vi "Untitled 1.vi"() -> ()   [LabVIEW 2019]
uses:
  <vilib>/Analysis/Matrix/NI_Matrix.lvlib
  <vilib>/Analysis/Matrix/Numeric/Add/Add - RM,RM.vi
  <vilib>/Analysis/Matrix/Datatypes/RealMatrix.ctl
panel:
  in  "Real Matrix 2":T1
  in  "Real Matrix":T1
  out "matrice":bool[][](array[boolean])
  in  "vect":dbl[](array[numeric])
  out "NB ITERATIONS":i32
  in  "STOP":bool
  out "x*y":dbl
  in  "stop":bool
  out "TE(ms)":u32
  out "TF(ms)":dbl
  out "IT(ms)":dbl
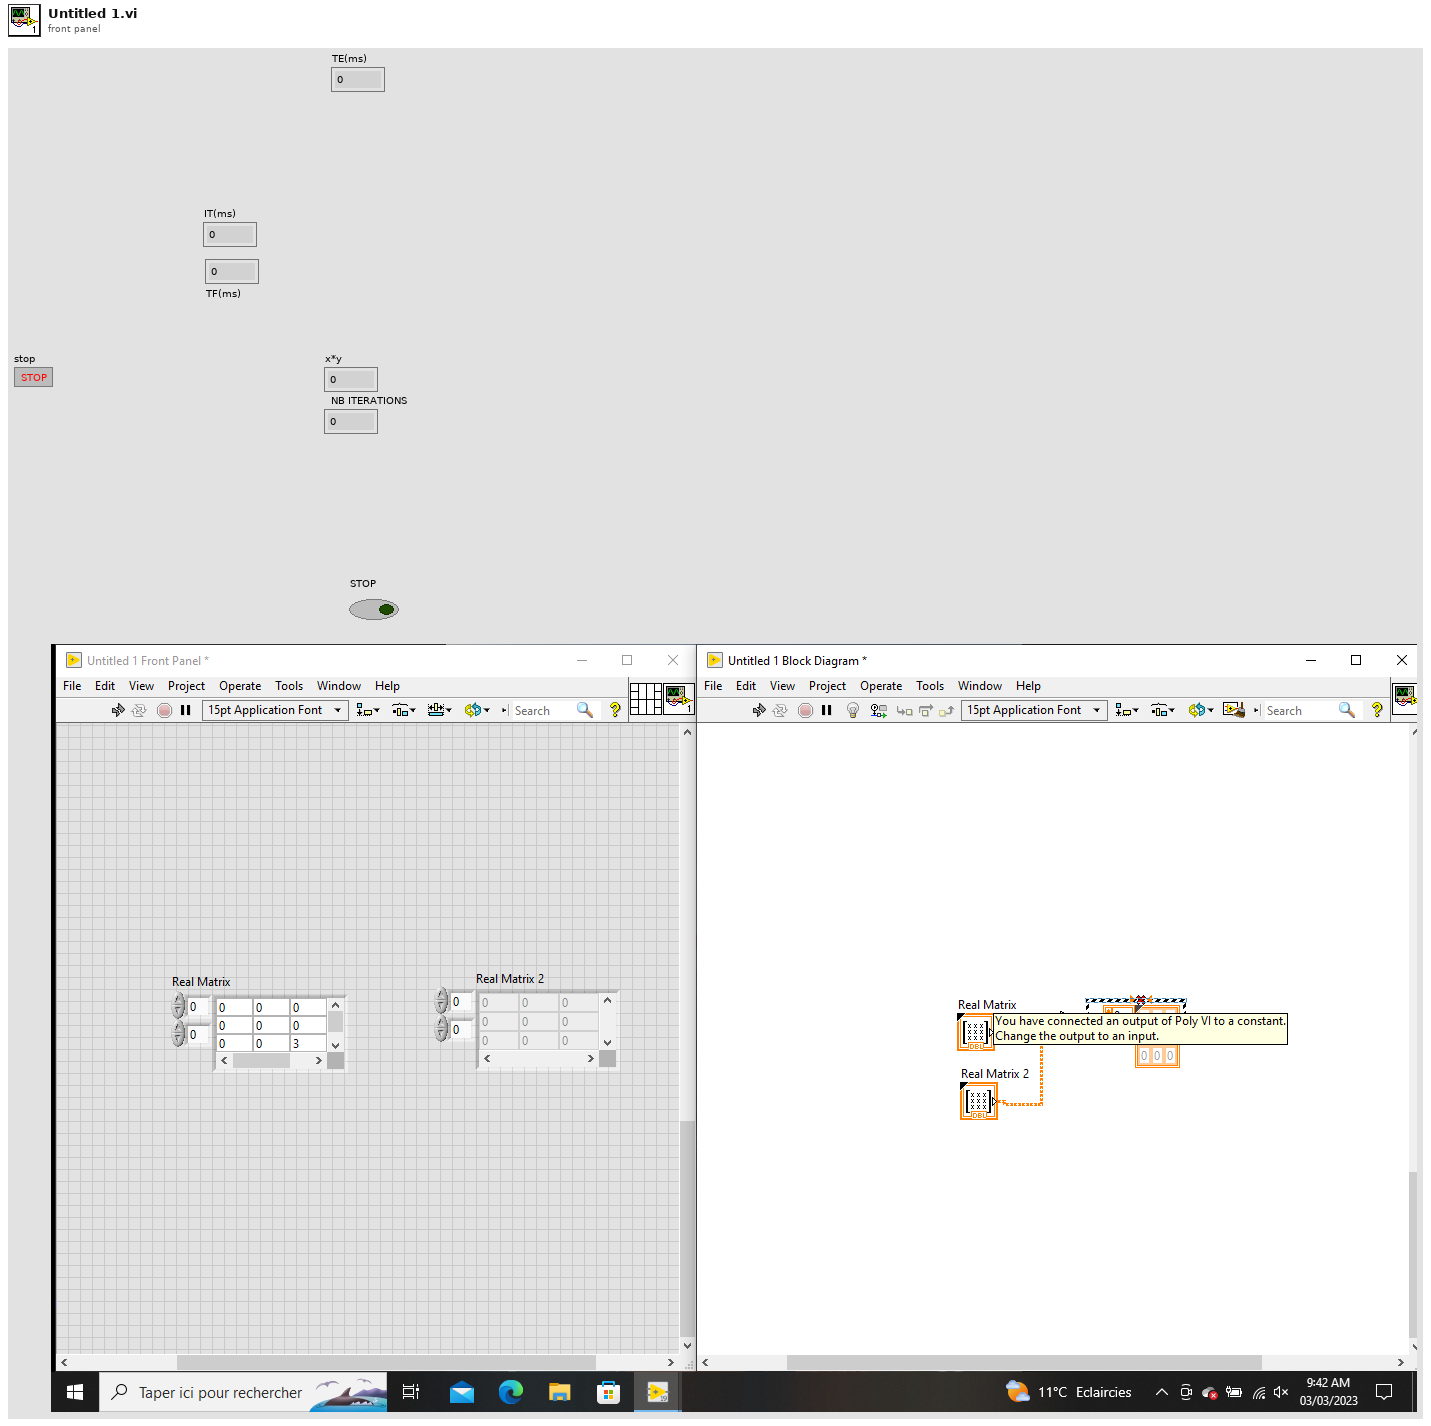
[diagram p1: front panel]
types:
  T1 = typedef "NI_Matrix.lvlib/RealMatrix.ctl" = dbl[][]
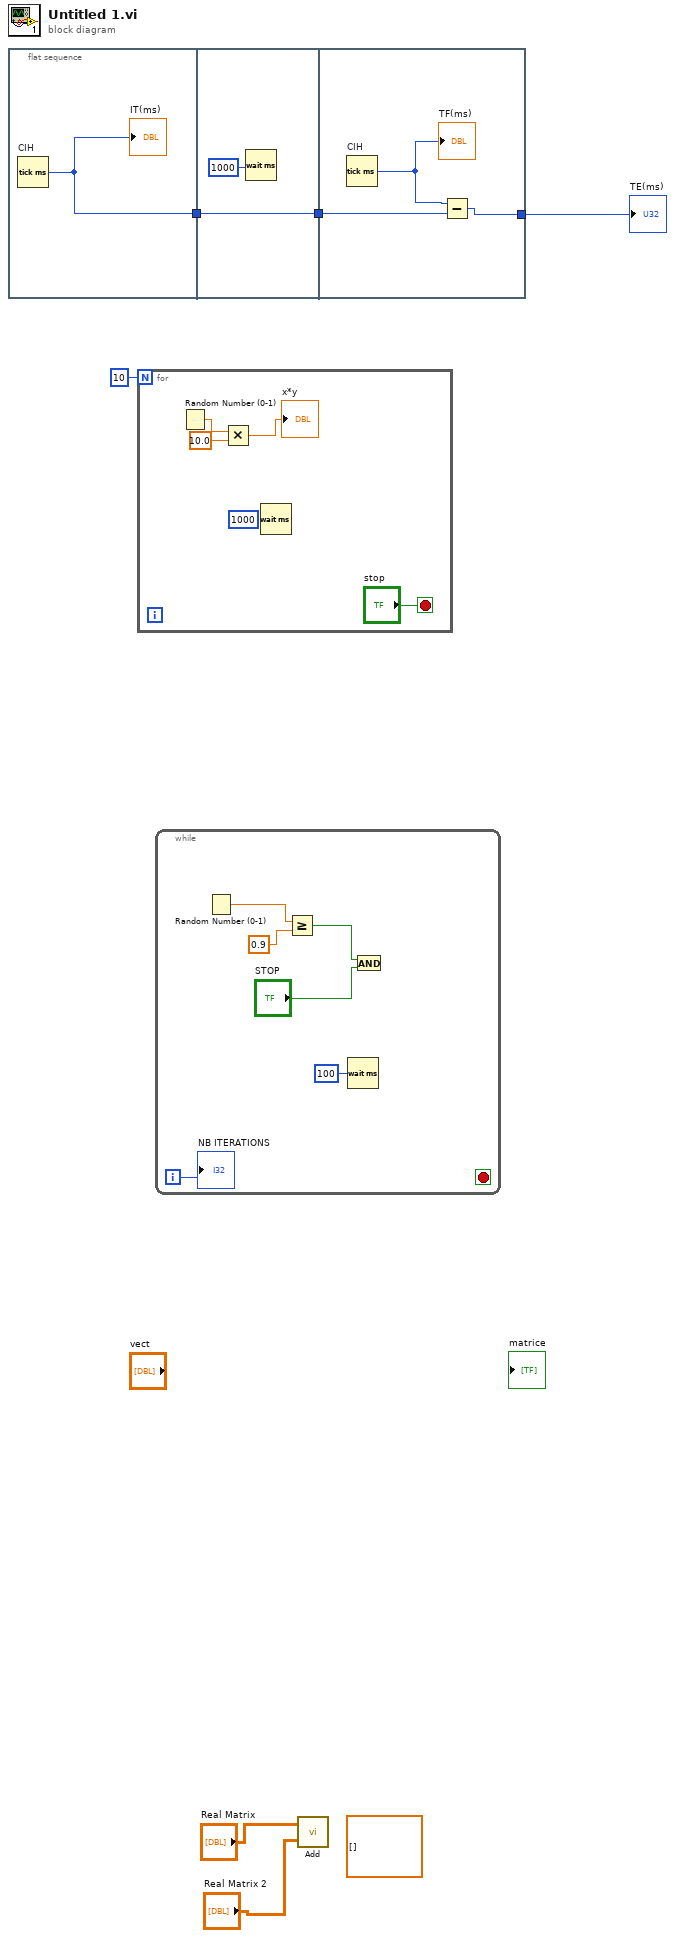
[diagram p0: block diagram]
diagram:
  (unwired) T1 [] ("Real Matrix B")
  n1 = flat-sequence {
    tunnel: [w7] -> w5
    tunnel: [w9] -> w6
    tunnel: w5 -> [w9]
    tunnel: w6 -> [w12]
    tunnel: [w10] -> w4
    frame #0 {
      n2 = Tick Count (ms) "CIH"() -> (millisecond timer value=w7:u32)
      "IT(ms)" <- w7
    }
    frame #1 {
      n3 = Wait (ms)(milliseconds to wait=u32 1000 ("millisecond timer value")) -> ()  [unwired: 1 out]
    }
    frame #2 {
      n4 = Tick Count (ms) "CIH"() -> (millisecond timer value=w11:u32)
      "TF(ms)" <- w11
      n5 = Subtract(x=w11, y=w12) -> (x-y=w10:u32)
    }
  }
  n6 = for {
    N: 10 -> [_]
    stop <- "stop" stop-if-true
    (unwired) u32 1000 ("millisecond timer value")
    n7 = Random Number (0-1)() -> (number: 0 to 1=w16:dbl)
    n8 = Multiply(x=w16, y=10.0) -> (x*y=→"x*y":dbl)
    n9 = Wait (ms)() -> ()  [unwired: 1 in, 1 out]
  }
  n10 = while {
    i -> [w20]
    stop <- _ stop-if-true
    n11 = Random Number (0-1)() -> (number: 0 to 1=w18:dbl)
    n12 = Greater Or Equal?(x=w18, y=0.9 ("x")) -> (x >= y?=w21:bool)
    n13 = Wait (ms)(milliseconds to wait=u32 100) -> ()  [unwired: 1 out]
    n14 = And(x=w21, y="STOP") -> ()  [unwired: 1 out]
    "NB ITERATIONS" <- w20
  }
  n15 = call-poly <vilib>:"Add.vi"("Real Matrix B"="Real Matrix 2", "Real Matrix A"="Real Matrix") -> ()  [unwired: 1 out]
  "TE(ms)" <- w4
